vi "RR asynchronous autofocus.vi"() -> ()   [LabVIEW 2011]
uses:
  Autofocus Globals.vi
panel:
  in  "Delay time (s)":dbl
  in  "Run?":bool
  # "WARNING: Do not run this program unless an appropriate filter \nis in place to protect the camera from the IR laser scatter.\n\nExit asynchronous autofocus by unchecking the \"Run continuously\" box.  Do\nnot exit by closing this window."
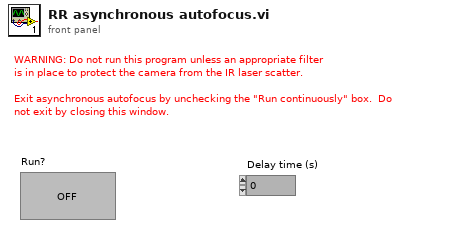
[diagram p1: front panel]
types:
  T1 = typedef "Laser type.ctt" = enum16{"Blue 488 nm", "Green 532 nm", "Red 633 nm", "IR 780"}
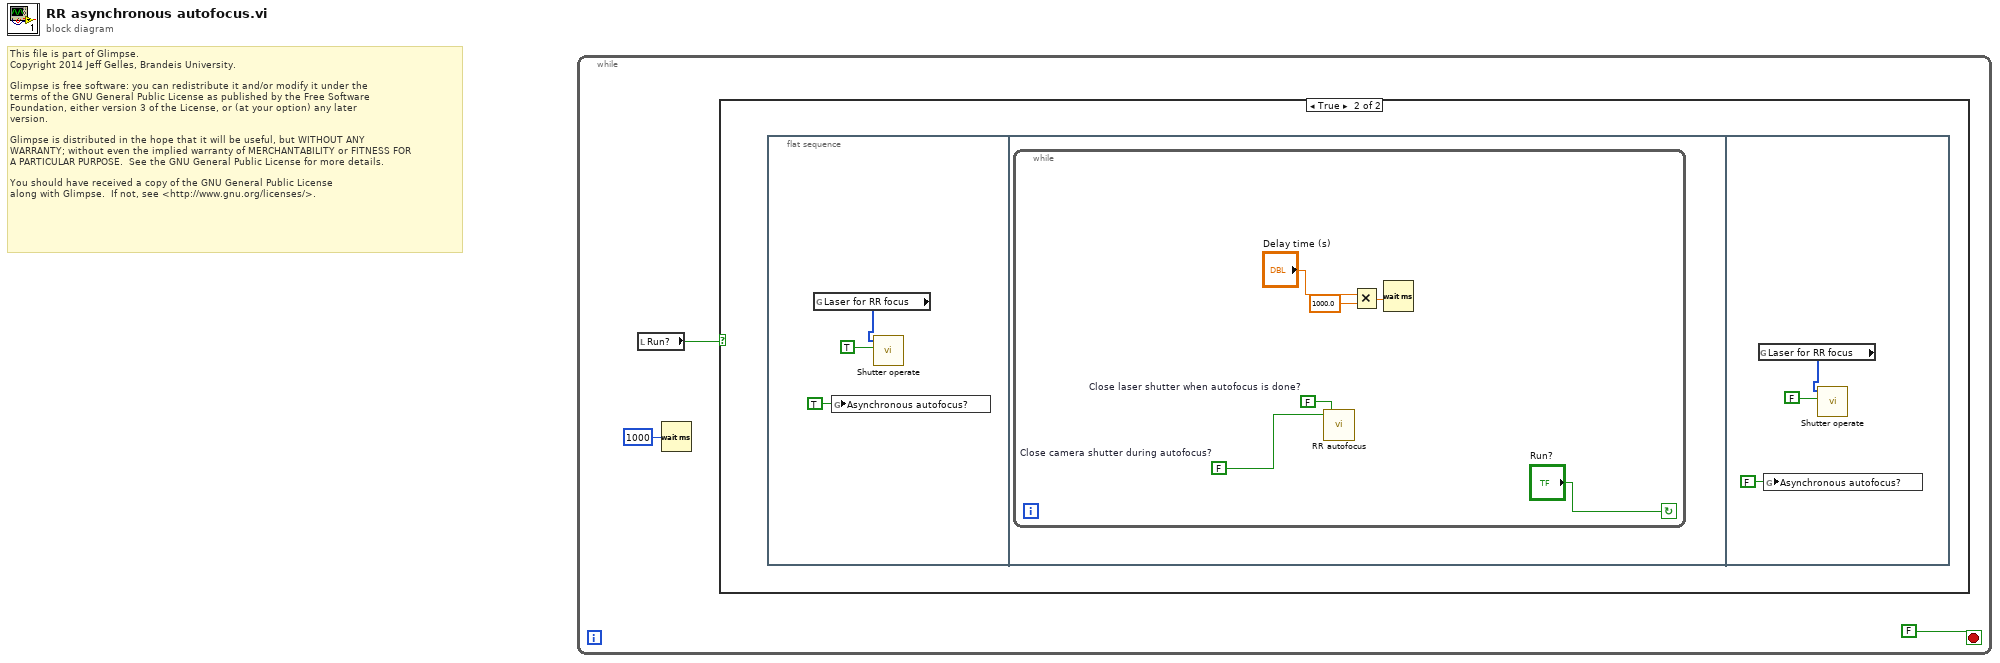
[diagram p0: block diagram]
diagram:
  # "This file is part of Glimpse. \nCopyright 2014 Jeff Gelles, Brandeis University.    \n\nGlimpse is free software: you can redistribute it and/or modify it under the \nterms of the GNU General Public License as published by the Free Software \nFoundation, either version 3 of the License, or (at your option) any later \nversion.\n\nGlimpse is distributed in the hope that it will be useful, but WITHOUT ANY \nWARRANTY; without even the implied warranty of MERCHANTABILITY or FITNESS FOR \nA PARTICULAR PURPOSE.  See the GNU General Public License for more details.\n\nYou should have received a copy of the GNU General Public License\nalong with Glimpse.  If not, see <http://www.gnu.org/licenses/>."
  n1 = while {
    stop <- FALSE ("stop") stop-if-true
    n2 = local read "Run?"() -> (w3:bool)
    n3 = Wait (ms)(milliseconds to wait=u32 1000) -> ()  [unwired: 1 out]
    n4 = case shown="True" w3 {
      frame False {
      }
      frame True {
        n5 = flat-sequence {
          frame #0 {
            n6 = global read "Autofocus Globals.vi" "Laser for RR focus"() -> (w5:T1[])
            n7 = global write "Autofocus Globals.vi" "Asynchronous autofocus?"(TRUE ("Asynchronous autofocus?")) -> ()
            n8 = call "Shutter operate.vi"("Shutters"=w5, 2:TRUE ("Data to Write")) -> ()  [unwired: 1 in, 6 out]
          }
          frame #1 {
            n9 = while {
              stop <- "Run?" continue-if-true
              w7 = FALSE  # Close laser shutter when autofocus is done?
              w11 = FALSE  # Close camera shutter during autofocus?
              n10 = call "RR autofocus.vi"("Close camera shutter during autofocus?"=w11, "Close laser shutter when autofocus is done?"=w7) -> ()  [unwired: 5 in, 1 out]
              n11 = Multiply(x="Delay time (s)", y=1000.0) -> (x*y=w10:dbl)
              n12 = Wait (ms)(milliseconds to wait=w10) -> ()  [unwired: 1 out]
            }
          }
          frame #2 {
            n13 = global read "Autofocus Globals.vi" "Laser for RR focus"() -> (w14:T1[])
            n14 = global write "Autofocus Globals.vi" "Asynchronous autofocus?"(FALSE ("Asynchronous autofocus?")) -> ()
            n15 = call "Shutter operate.vi"("Shutters"=w14, 2:FALSE ("Data to Write")) -> ()  [unwired: 1 in, 6 out]
          }
        }
      }
    }
  }
